vi "Modbus_Slave.vi"() -> ()   [LabVIEW 2020]
uses:
  <vilib>/NI/Modbus Library/API/Wrapper/Create TCP Slave.vi
  <vilib>/NI/Modbus Library/API/Slave/Modbus Slave.lvclass
  <vilib>/NI/Modbus Library/API/Wrapper/API Main.lvlib
panel:
  out "Array 2":bool[](array[boolean])
  in  "number of inputs 2":u16
  in  "starting address 2":u16
  out "Array":bool[](array[boolean])
  in  "number of inputs":u16
  in  "starting address":u16
  in  "stop":bool
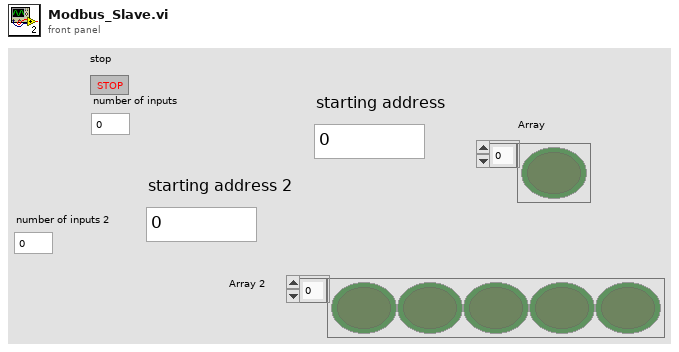
[diagram p1: front panel]
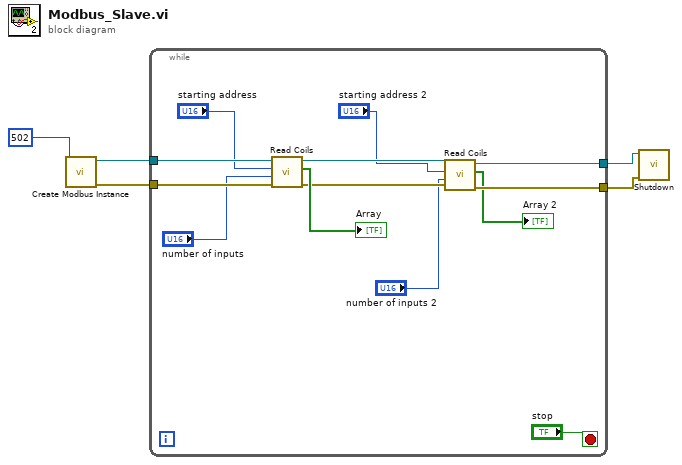
[diagram p0: block diagram]
diagram:
  n1 = call-poly <vilib>:"Create Modbus Instance.vi"("port (502)"=u16 502) -> ("error out"=w3:errorcluster, "TCP slave instance"=w4:refnum<class "Modbus Slave.lvclass">)  [unwired: 9 in]
  n2 = while {
    tunnel: w4 -> [w17]
    tunnel: w3 -> [w16]
    tunnel: [w8] -> w2
    tunnel: [w7] -> w1
    stop <- "stop" stop-if-true
    n3 = call-dynamic "Read Coils.vi"("error in"=w16, "number of inputs"="number of inputs", "starting address"="starting address", "Modbus slave in"=w17) -> ("error out"=w11:errorcluster, "coils"=→"Array":bool[], "Modbus slave out"=w12:refnum<class "Modbus Slave.lvclass">)  [unwired: 5 in]
    n4 = call-dynamic "Read Coils.vi"("error in"=w11, "number of inputs"="number of inputs 2", "starting address"="starting address 2", "Modbus slave in"=w12) -> ("error out"=w7:errorcluster, "coils"=→"Array 2":bool[], "Modbus slave out"=w8:refnum<class "Modbus Slave.lvclass">)  [unwired: 5 in]
  }
  n5 = call-dynamic "Shutdown.vi"("error in"=w1, "Modbus slave in"=w2) -> ()  [unwired: 9 in, 1 out]
